vi "process-booleans.vi"(10 "boolean indicators 2":T1) -> (0 "scaning finished":bool, 2 "boolean indicators":T1)   [LabVIEW 2017]
uses:
  controls/boolean_info.ctl
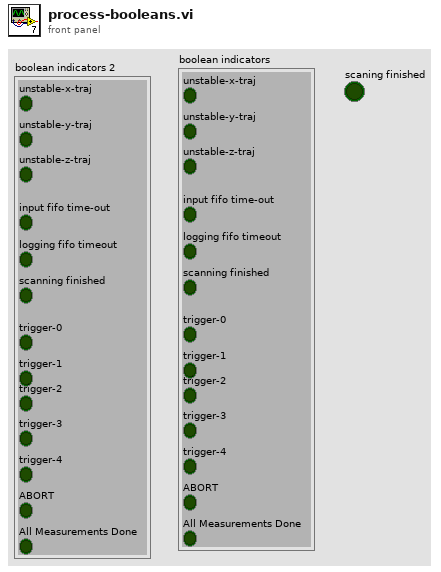
[diagram p1: front panel]
types:
  T1 = typedef "boolean_info.ctl" = cluster{"unstable-z-traj":bool, "input fifo time-out":bool, "logging fifo timeout":bool, "scanning finished":bool, "trigger-1":bool, "trigger-0":bool, "trigger-2":bool, "trigger-3":bool, "trigger-4":bool, "unstable-x-traj":bool, "unstable-y-traj":bool, "ABORT":bool, "All Measurements Done":bool}
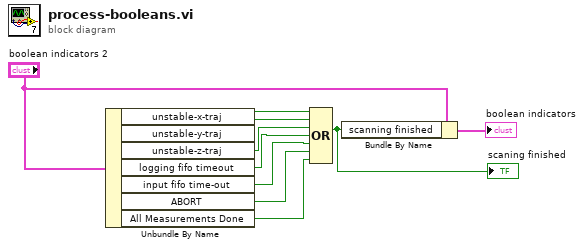
[diagram p0: block diagram]
diagram:
  n1 = Unbundle By Name("boolean indicators 2") -> ("unstable-x-traj"=w10:bool, "unstable-y-traj"=w9:bool, "unstable-z-traj"=w8:bool, "logging fifo timeout"=w7:bool, "input fifo time-out"=w6:bool, "ABORT"=w5:bool, "All Measurements Done"=w1:bool)
  n2 = Compound Arithmetic op=OR(w10, w9, w8, w7, w6, w5, w1) -> (w4:bool)
  "scaning finished" <- w4
  n3 = Bundle By Name(cluster="boolean indicators 2", "scanning finished"=w4) -> (→"boolean indicators":T1)
